vi "GetVIReference.vi"(8 "error in (no error)":errorcluster, 10 "vi type":T2(ring), 11 "file path":path) -> (0 "error out":errorcluster, 3 "reference out":refnum<vi>)   [LabVIEW 2013]
doc: "This VI creates a new file or open the reference if the file already exists"
uses:
  Controls/PathsCluster.ctl
panel:
  in  "Paths":T1
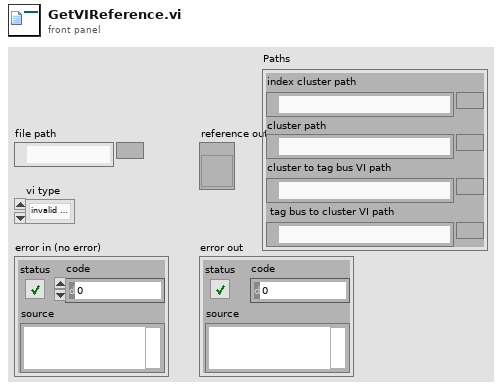
[diagram p1: front panel]
types:
  T1 = typedef "PathsCluster.ctl" = cluster{"index cluster path":path, "cluster path":path, "cluster to tag bus VI path":path, " tag bus to cluster VI path":path}
  T2 = enum32{"invalid VI type", "Standard VI", "Control VI", "Global VI", "Polymorphic VI", "Configuration VI", "SubSystem", "Facade VI", "Method VI"}
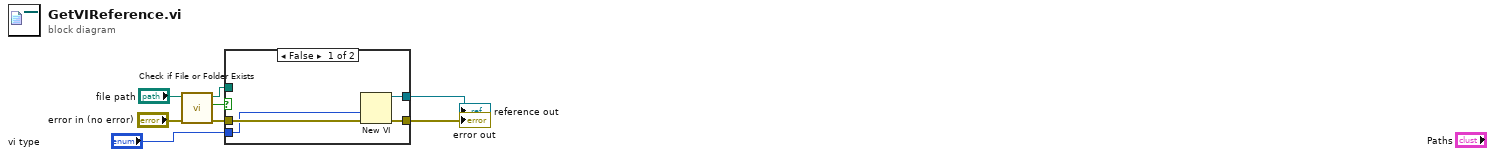
[diagram p0: block diagram]
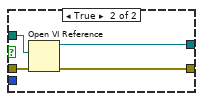
[diagram p2: hidden frame]
diagram:
  n1 = call <vilib>:"Check if File or Folder Exists.vi"("error in (no error)"="error in (no error)", "path"="file path") -> ("error out"=w4:errorcluster, "file or folder exists?"=w5:bool, "dup path"=w6:path)  [unwired: 7 in]
  n2 = case shown="False" w5 {
    tunnel: [w12 w14] -> w1
    tunnel: w4 -> [w11 w15]
    tunnel: w6 -> [_ w16]
    tunnel: [w10 w13] -> w7
    tunnel: "vi type" -> [w9 _]
    frame False {
      n3 = New VI(8:w11, 9:w9) -> (0:w10:errorcluster, 3:w12:refnum<vi>)  [unwired: 5 out]
    }
    frame True {
      n4 = Open VI Reference(vi path=w16, error in (no error)=w15) -> (vi reference=w14:refnum<vi>, error out=w13:errorcluster)  [unwired: 4 in]
    }
  }
  "error out" <- w7
  "reference out" <- w1
